vi "Set Global StateType Filter.vi"(10 "Group:LogType":T1[](array[typedef]), 11 "GlobalLogFilter in":refnum<class "LogFilter.lvclass">) -> (3 "GlobalLogFilter out":refnum<class "LogFilter.lvclass">)   [LabVIEW 2020, in "Communicable State Machine.lvlib" / "LogFilter.lvclass"]
uses:
  LogFilter.lvclass
  _CSM_GlobalLog_STATE_TYPE.ctl
  LogFilter.lvclass/LogFilter.ctl
  Communicable State Machine.lvlib
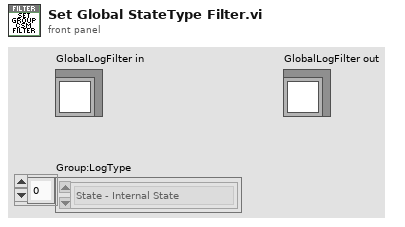
[diagram p1: front panel]
types:
  T1 = typedef "Communicable State Machine.lvlib/_CSM_GlobalLog_STATE_TYPE.ctl" = enum16{"State - Internal State", "State - External Message", "State - Response", "State - Complete"}
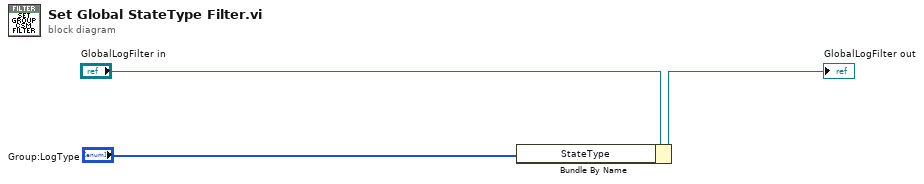
[diagram p0: block diagram]
diagram:
  n1 = Bundle By Name(cluster="GlobalLogFilter in", "StateType"="Group:LogType") -> (→"GlobalLogFilter out":refnum<class "LogFilter.lvclass">)
